vi "FileIOByBinary.vi"() -> ()   [LabVIEW 2021]
panel:
  out "data":string
  out "I32read":i32
  out "DBLread":dbl
  in  "String":string
  in  "I32":i32
  in  "DBL":dbl
  in  "Write":bool
  in  "file path (use dialog)":path
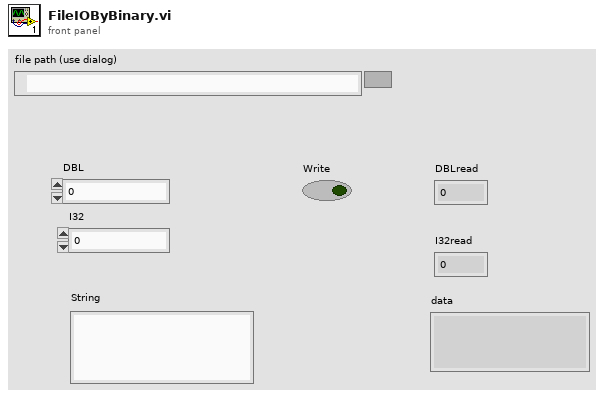
[diagram p1: front panel]
types:
  T1 = enum16{"big-endian, network order", "native, host order", "little-endian"}
  T2 = enum16{"open", "replace", "create", "open or create", "replace or create", "replace or create with confirmation"}
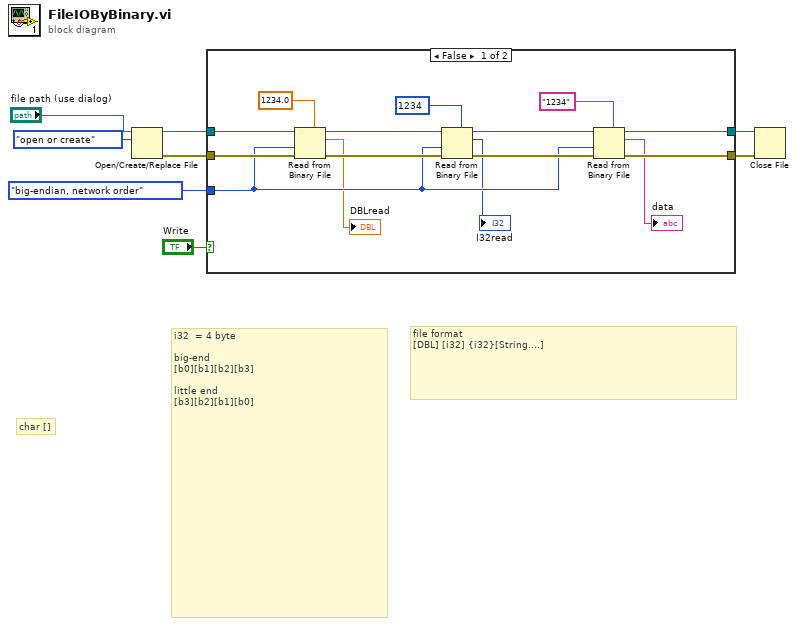
[diagram p0: block diagram]
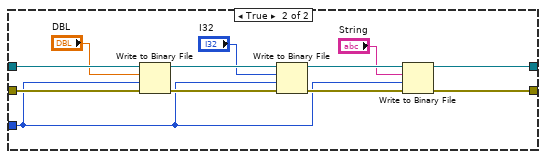
[diagram p2: hidden frame]
diagram:
  # "char []"
  # "i32  = 4 byte \n\nbig-end\n[b0][b1][b2][b3]\n\nlittle end \n[b3][b2][b1][b0]"
  # "file format \n[DBL] [i32] {i32}[String....]"
  n1 = Open/Create/Replace File(file path (use dialog)="file path (use dialog)", operation (0:open)=T2."open or create") -> (refnum out=w8:refnum<file>, error out=w7:errorcluster)  [unwired: 4 in, 1 out]
  n2 = case shown="False" "Write" {
    tunnel: w8 -> [w23 w33]
    tunnel: w7 -> [w22 w35]
    tunnel: [w16 w28] -> w6
    tunnel: [w17 w30] -> w5
    tunnel: T1."big-endian, network order" ("byte order (0:big-endian, network order)") -> [w12 w24]
    frame False {
      n3 = Read from Binary File(5:1234.0 ("DBL"), 8:w22, 9:w12, 11:w23) -> (0:w20:errorcluster, 2:→"DBLread":dbl, 3:w21:refnum<file>)  [unwired: 2 in, 1 out]
      n4 = Read from Binary File(5:1234 ("I32"), 8:w20, 9:w12, 11:w21) -> (0:w18:errorcluster, 2:→"I32read":i32, 3:w19:refnum<file>)  [unwired: 2 in, 1 out]
      n5 = Read from Binary File(5:"1234" ("String"), 8:w18, 9:w12, 11:w19) -> (0:w17:errorcluster, 2:→"data":string, 3:w16:refnum<file>)  [unwired: 2 in, 1 out]
    }
    frame True {
      n6 = Write to Binary File(file (use dialog)=w33, data="DBL", error in=w35, 9:w24) -> (refnum out=w31:refnum<file>, error out=w34:errorcluster)  [unwired: 2 in, 1 out]
      n7 = Write to Binary File(file (use dialog)=w31, data="I32", error in=w34, 9:w24) -> (refnum out=w29:refnum<file>, error out=w32:errorcluster)  [unwired: 2 in, 1 out]
      n8 = Write to Binary File(file (use dialog)=w29, data="String", error in=w32, 9:w24) -> (refnum out=w28:refnum<file>, error out=w30:errorcluster)  [unwired: 2 in, 1 out]
    }
  }
  n9 = Close File(refnum=w6, error in=w5) -> ()  [unwired: 2 out]
